vi "virtualinstrument.vi"() -> ()   [LabVIEW 2025]
uses:
  <vilib>/httpClient/LabVIEWHTTPClient.lvlib
  <extravilib>/ChannelInstances/Tag-bool.lvlib
  <vilib>/regexp/Match Regular Expression.xnode
  <vilib>/httpClient/POSTBuffer.vi
  <vilib>/Instr/_visa.llb/VISA Configure Serial Port (Instr).vi
panel:
  out "indexminim":i32
  out "indexmax":i32
  out "humarray":dbl[](array[numeric])
  out "temparray":dbl[](array[numeric])
  out "ppmarray":dbl[](array[numeric])
  out "<JSON>":string[](array[string]) caption="<JSON>Elements"
  in  "Tab Control":enum32{"Page 1"}(tab)
  in  "Select interval":bool
  in  "min":string(combo)
  out "Waveform Chart":dbl[](graph) caption="PPM CHART"
  in  "Select":enum16{"hum", "temp", "ppm"}(ring)
  out "Umiditate":dbl(knob) scale=0.0..100.0
  out "Temperatura":dbl(slide) caption="Thermometer" scale=0.0..100.0
  in  "stop":bool
  in  "Enum":enum16{"PPM", "TEMP", "HUM"}(ring)
  in  "interval \nmasurare[s]":u32=1
  out "XY Graph":cluster{"array":u32[], dbl[]}(graph) caption="PPM GRAPH"
  in  "interval \ntrimitere[s]":u32=1
  out "error out":errorcluster
  out "read buffer":string
  out "ppm":u32(colorbox)
  out "confort termic":dbl
  out "heat index":dbl
  out "ppm":dbl
  in  "Get data from \nspreadsheet":bool
  out "datesarray":timestamp[](array[timestamp]) format="%<%H:%M:%S\n%x>T"
  out "max value":timestamp format="%<%H:%M:%S\n%x>T"
  out "min value":timestamp format="%<%H:%M:%S\n%x>T"
  in  "max":string(combo)
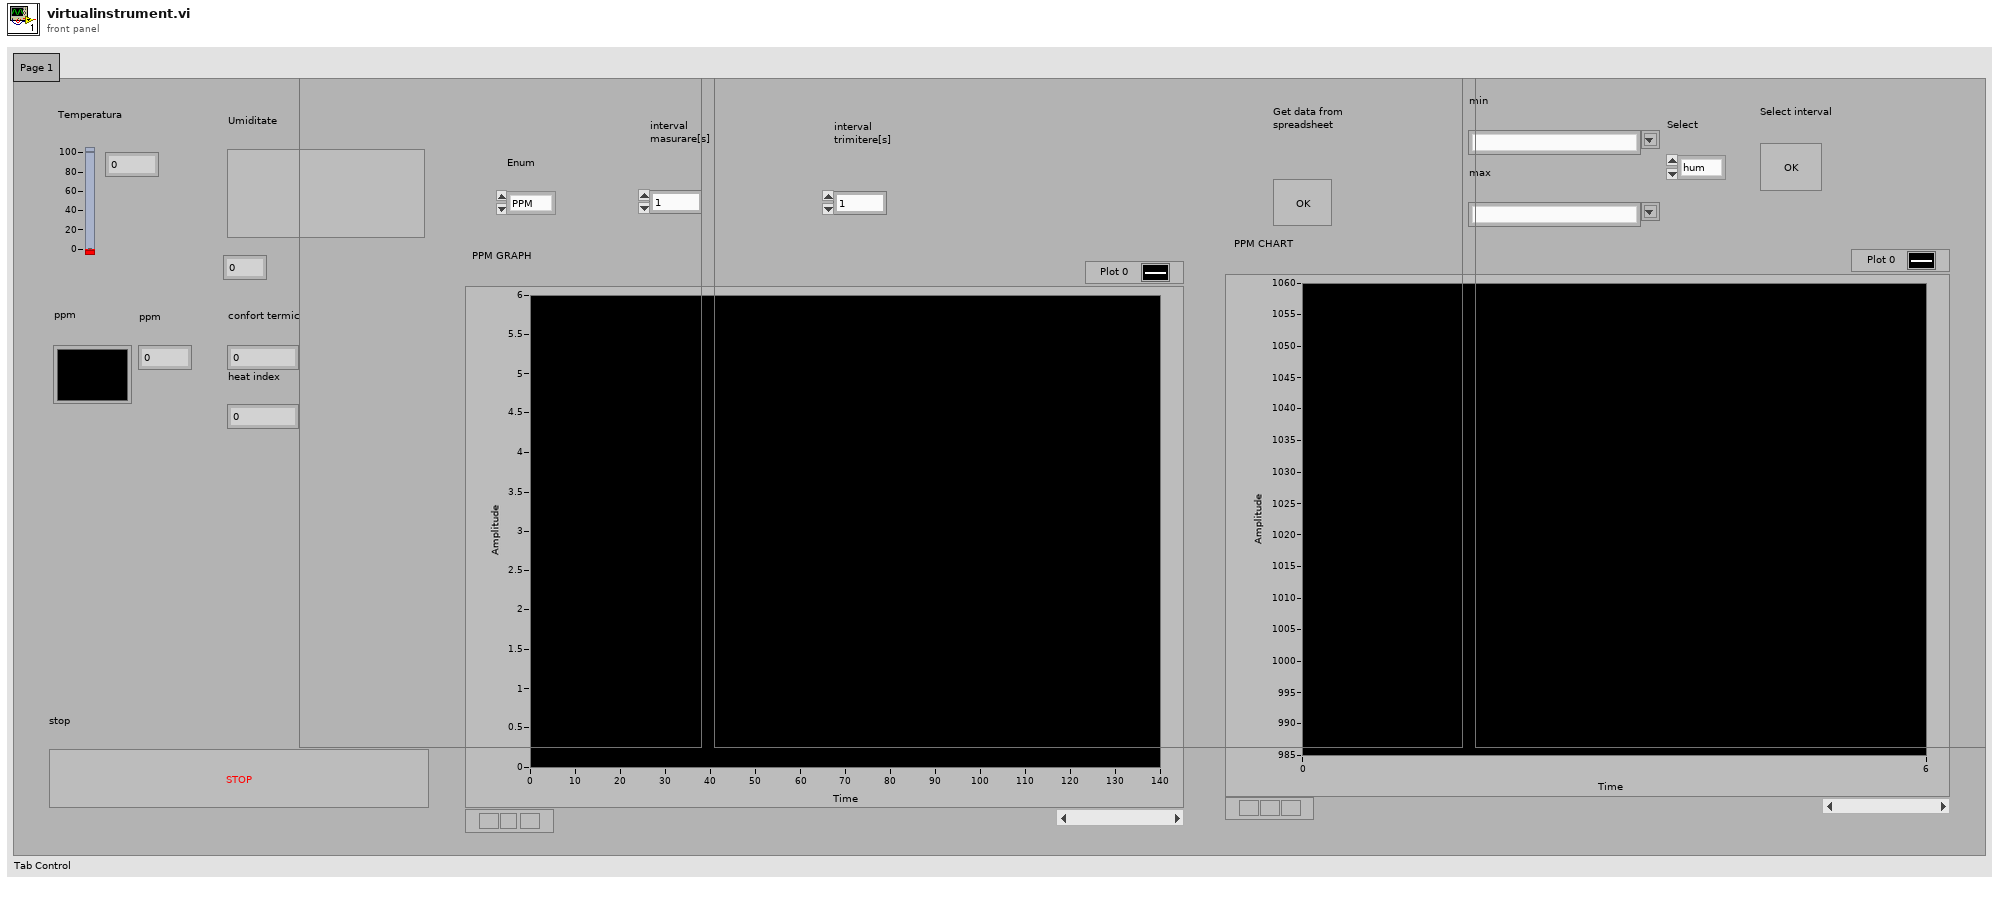
[diagram p1: front panel]
types:
  T1 = typedef "Tag-bool.lvlib/))Channel.ctl" = refnum<queue>
  T2 = enum8{"Enabled", "Disabled", "Disabled and Grayed Out"}
  T3 = typedef "LabVIEWHTTPClient.lvlib/ClientHandle.ctl" = refnum<k1>
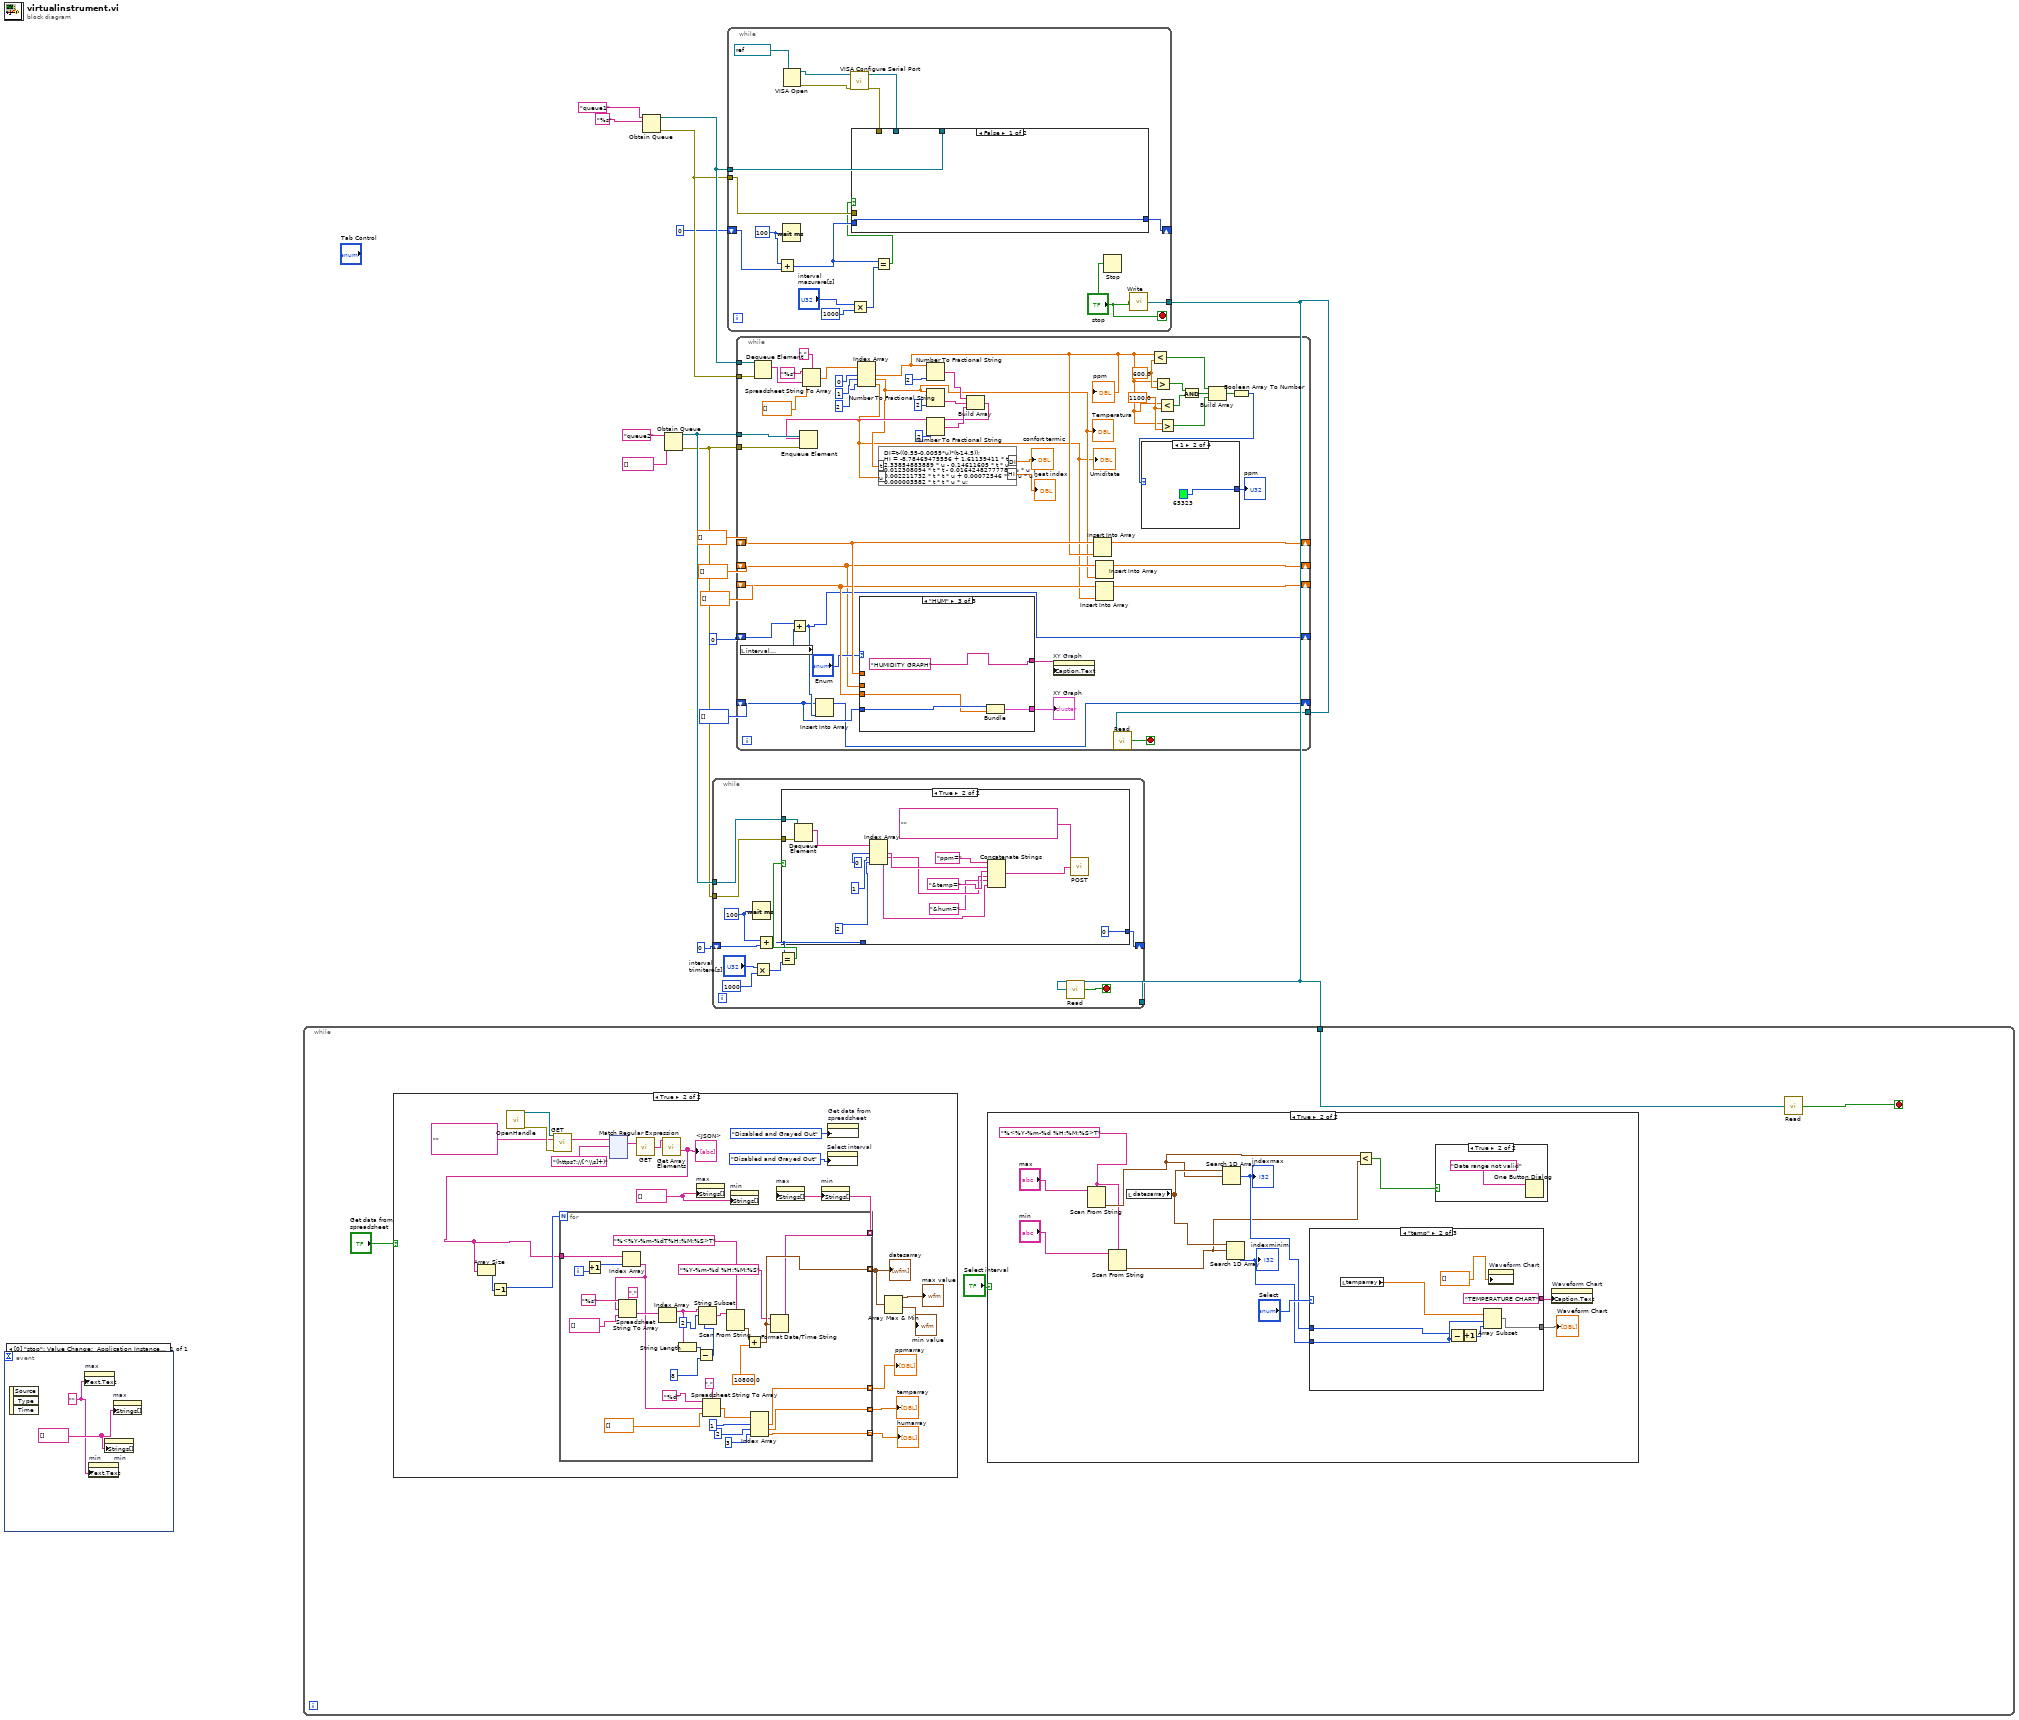
[diagram p0: block diagram]
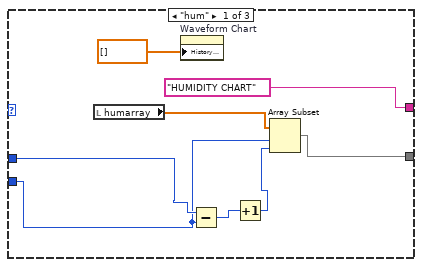
[diagram p3: hidden frame]
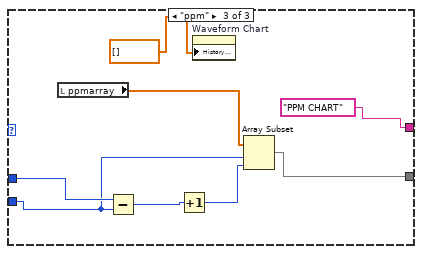
[diagram p4: hidden frame]
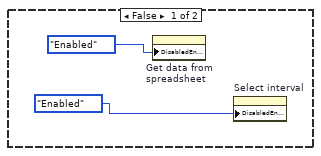
[diagram p6: hidden frame]
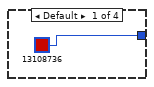
[diagram p8: hidden frame]
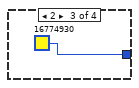
[diagram p9: hidden frame]
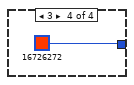
[diagram p10: hidden frame]
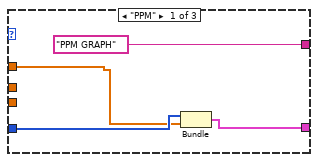
[diagram p11: hidden frame]
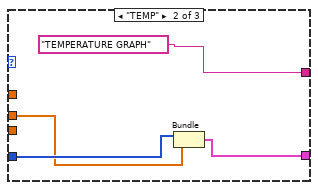
[diagram p12: hidden frame]
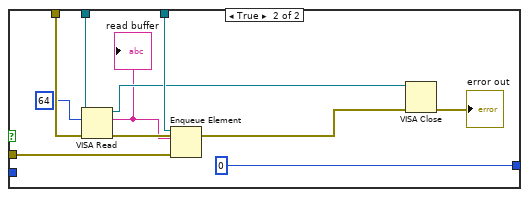
[diagram p13: hidden frame]
diagram:
  n1 = event shown="[0] \"stop\": Value Change;  Application Instance Close" {
    selector: _ -> [_]
    dyn-events: _ -> [_]
    timeout: _ -> [_]
    event "stop": Value Change; Application Instance Close {
      w17 = "" ("Text.Text")
      w18 = string[] []
      n2 = event-data() -> ()  [unwired: 1 in, 3 out]
      n3 = property on="max" class="CmbBox"("Text.Text"=w17) -> ()  [unwired: 2 in, 2 out]
      n4 = property on="min" class="CmbBox"("Text.Text"=w17) -> ()  [unwired: 2 in, 2 out]
      n5 = property on="min" class="CmbBox"("Strings[]"=w18) -> ()  [unwired: 2 in, 2 out]
      n6 = property on="max" class="CmbBox"("Strings[]"=w18) -> ()  [unwired: 2 in, 2 out]
    }
  }
  n7 = Obtain Queue(name (unnamed)="queue1", element data type="%s") -> (queue out=w7:refnum<queue>, error out=w6:errorcluster)  [unwired: 3 in, 1 out]
  n8 = Obtain Queue(name (unnamed)="queue2", element data type=string[] []) -> (queue out=w12:refnum<queue>, error out=w11:errorcluster)  [unwired: 3 in, 1 out]
  n9 = while {
    tunnel: [w35] -> w1
    tunnel: w7 -> [w28]
    tunnel: w6 -> [w27]
    shift-right: [w29] -> _
    shift-left: u32 0 ("y") -> [w26]
    stop <- "stop" stop-if-true
    w30 = u32 100 ("y")
    n10 = Add(x=w30, y=w26) -> (x+y=w22:u32)
    n11 = Wait (ms)(milliseconds to wait=w30) -> ()  [unwired: 1 out]
    n12 = VISA Open(VISA resource name=refnum<visa-resource-name> "COM3") -> (VISA resource name=w33:refnum<visa-resource-name>, error out=w34:errorcluster)  [unwired: 4 in]
    n13 = call-poly "VISA Configure Serial Port"("VISA resource name"=w33, "error in (no error)"=w34) -> ("VISA resource name out"=w19:refnum<visa-resource-name>, "error out"=w20:errorcluster)  [unwired: 12 in]
    n14 = Multiply(x="interval \nmasurare[s]", y=u32 1000) -> (x*y=w23:u32)
    n15 = Equal?(x=w22, y=w23) -> (x = y?=w21:bool)
    n16 = case shown="False" w21 {
      tunnel: [w36 u32 0 ("y")] -> w29
      tunnel: w28 -> [_ w45]
      tunnel: w27 -> [_ w44]
      tunnel: w22 -> [w36 _]
      tunnel: w20 -> [_ w40]
      tunnel: w19 -> [_ w39]
      frame False {
      }
      frame True {
        n17 = VISA Read(VISA resource name=w39, byte count=u32 64, error in (no error)=w40) -> (VISA resource name out=w43:refnum<visa-resource-name>, read buffer=w38:string, error out=w42:errorcluster)  [unwired: 1 out]
        "read buffer" <- w38
        n18 = Enqueue Element(queue=w45, element=w38, error in (no error)=w44) -> ()  [unwired: 1 in, 3 out]
        n19 = VISA Close(VISA resource name=w43, error in (no error)=w42) -> (error out=→"error out":errorcluster)
      }
    }
    n20 = Stop(stop? (T)="stop") -> ()
    n21 = call <extravilib>:"Write.vi"("element"="stop") -> ("channel"=w35:T1)  [unwired: 1 out]
  }
  n22 = while {
    tunnel: w1 -> [w50]
    stop <- w49 stop-if-true
    n23 = case shown="True" "Get data from \nspreadsheet" {
      frame False {
        n24 = property on="Get data from \nspreadsheet" class="Bool"("DisabledEnum"=T2."Enabled" ("Disabled")) -> ()  [unwired: 2 in, 2 out]
        n25 = property on="Select interval" class="Bool"("DisabledEnum"=T2."Enabled" ("Disabled")) -> ()  [unwired: 2 in, 2 out]
      }
      frame True {
        w92 = string[] []
        n26 = call <vilib>:"OpenHandle.vi"() -> ("client handle out"=w109:T3, "error out"=w108:errorcluster)  [unwired: 14 in]
        n27 = call <vilib>:"GET.vi"("client handle"=w109, "url"="", "error in (no error)"=w108) -> ("headers"=w105:string)  [unwired: 9 in, 3 out]
        n28 = xnode ("Match Regular Expression")("input string"=w105, "regular expression"="(https?://[^\\s]+)") -> ("whole match"=w90:string)  [unwired: 4 in, 4 out]
        n29 = call <vilib>:"GET.vi"("url"=w90) -> ("body"=w104:string)  [unwired: 11 in, 3 out]
        n30 = call <vilib>:"Get Array Elements.vi"("JSON"=w104) -> ("<JSON>"=w94:string[])  [unwired: 8 in, 2 out]
        "<JSON>" <- w94
        n31 = Array Size(array=w94) -> (size(s)=w100:i32)
        n32 = Decrement(x=w100) -> (x-1=w99:i32)
        n33 = for {
          N: w99 -> [_]
          tunnel: w94 -> [w138]
          tunnel: [w130] -> w101 mode=indexing
          tunnel: [w120] -> w103 mode=indexing
          tunnel: [w119] -> w102 mode=indexing
          tunnel: [w114] -> w98 mode=indexing
          tunnel: [w110] -> w93 mode=indexing
          i -> [w139]
          n34 = Increment(x=w139) -> (x+1=w133:i32)
          n35 = Index Array(array=w138, index=w133) -> (element=w118:string)
          n36 = Spreadsheet String To Array(delimiter (Tab)=",", format string="%s" ("delimiter (Tab)"), spreadsheet string=w118, array type (2D Dbl)=string[] []) -> (array=w136:string[])
          n37 = Index Array(array=w136) -> (element=w126:string)  [unwired: 1 in]
          n38 = String Length(string=w126) -> (length=w125:i32)
          n39 = Subtract(x=w125, y=8) -> (x-y=w123:i32)
          n40 = String Subset(string=w126, offset (0)=2, length (rest)=w123) -> (substring=w113:string)
          n41 = Spreadsheet String To Array(delimiter (Tab)=",", format string="%d", spreadsheet string=w118, array type (2D Dbl)=dbl[] []) -> (array=w128:dbl[])
          n42 = Scan From String(format string="%<%Y-%m-%dT%H:%M:%S>T", input string=w113) -> (output 1=w115:timestamp)  [unwired: 3 in, 3 out]
          n43 = Add(x=w115, y=10800.0) -> (x+y=w114:timestamp)
          n44 = Index Array(array=w128, index #1=1 ("index"), index #2=2 ("index"), index #3=3 ("index")) -> (element #1=w130:dbl, element #2=w120:dbl, element #3=w119:dbl)
          n45 = Format Date/Time String(time format string (%c)="%Y-%m-%d %H:%M:%S", seconds (now)=w114) -> (date/time string=w110:string)  [unwired: 1 in]
        }
        "ppmarray" <- w101
        "temparray" <- w103
        "humarray" <- w102
        "datesarray" <- w98
        n46 = property on="max" class="CmbBox"("Strings[]"=w92) -> ()  [unwired: 2 in, 2 out]
        n47 = property on="min" class="CmbBox"("Strings[]"=w92) -> ()  [unwired: 2 in, 2 out]
        n48 = property on="max" class="CmbBox"("Strings[]"=w93) -> ()  [unwired: 2 in, 2 out]
        n49 = property on="min" class="CmbBox"("Strings[]"=w93) -> ()  [unwired: 2 in, 2 out]
        n50 = property on="Select interval" class="Bool"("DisabledEnum"=T2."Disabled and Grayed Out" ("Disabled")) -> ()  [unwired: 2 in, 2 out]
        n51 = property on="Get data from \nspreadsheet" class="Bool"("DisabledEnum"=T2."Disabled and Grayed Out" ("Disabled")) -> ()  [unwired: 2 in, 2 out]
        n52 = Array Max & Min(array=w98) -> (max value=→"max value":timestamp, min value=→"min value":timestamp)  [unwired: 2 out]
      }
    }
    n53 = case shown="True" "Select interval" {
      frame False {
      }
      frame True {
        w54 = "%<%Y-%m-%d %H:%M:%S>T" ("format string")
        n54 = Scan From String(format string=w54, input string="max") -> (output 1=w57:timestamp)  [unwired: 3 in, 3 out]
        n55 = Scan From String(format string=w54, input string="min") -> (output 1=w53:timestamp)  [unwired: 3 in, 3 out]
        n56 = local read "datesarray"() -> (w60:timestamp[])
        n57 = Search 1D Array(1D array=w60, element=w57) -> (index of element=w59:i32)  [unwired: 1 in]
        "indexmax" <- w59
        n58 = Search 1D Array(1D array=w60, element=w53) -> (index of element=w58:i32)  [unwired: 1 in]
        "indexminim" <- w58
        n59 = case shown="\"temp\"" "Select" {
          tunnel: w58 -> [w66 w75 w79]
          tunnel: w59 -> [w67 w74 w82]
          tunnel: [w65 w73 w83] -> w61
          tunnel: ["HUMIDITY CHART" ("Caption.Text") "TEMPERATURE CHART" ("Caption.Text") "PPM CHART" ("Caption.Text")] -> w51
          frame "hum" {
            n60 = local read "humarray"() -> (w70:dbl[])
            n61 = property on="Waveform Chart" class="WFChart (strict)"("History Data"=dbl[] []) -> ()  [unwired: 2 in, 2 out]
            n62 = Subtract(x=w67, y=w66) -> (x-y=w69:i32)
            n63 = Increment(x=w69) -> (x+1=w68:i32)
            n64 = Array Subset(array=w70, index=w66, length=w68) -> (w65:dbl[])
          }
          frame "temp" {
            n65 = local read "temparray"() -> (w78:dbl[])
            n66 = Subtract(x=w74, y=w75) -> (x-y=w77:i32)
            n67 = Increment(x=w77) -> (x+1=w76:i32)
            n68 = Array Subset(array=w78, index=w75, length=w76) -> (w73:dbl[])
            n69 = property on="Waveform Chart" class="WFChart (strict)"("History Data"=dbl[] []) -> ()  [unwired: 2 in, 2 out]
          }
          frame "ppm" {
            n70 = local read "ppmarray"() -> (w86:dbl[])
            n71 = Subtract(x=w82, y=w79) -> (x-y=w85:i32)
            n72 = Increment(x=w85) -> (x+1=w84:i32)
            n73 = property on="Waveform Chart" class="WFChart (strict)"("History Data"=dbl[] []) -> ()  [unwired: 2 in, 2 out]
            n74 = Array Subset(array=w86, index=w79, length=w84) -> (w83:dbl[])
          }
        }
        "Waveform Chart" <- w61
        n75 = Less?(x=w57, y=w53) -> (x < y?=w52:bool)
        n76 = case shown="True" w52 {
          frame False {
          }
          frame True {
            n77 = One Button Dialog(message="Date range not valid") -> ()  [unwired: 1 in, 1 out]
          }
        }
        n78 = property on="Waveform Chart" class="WFChart (strict)"("Caption.Text"=w51) -> ()  [unwired: 2 in, 2 out]
      }
    }
    n79 = call <extravilib>:"Read.vi"("channel"=w50) -> ("element"=w49:bool)  [unwired: 1 in, 1 out]
  }
  n80 = while {
    tunnel: w12 -> [w258]
    tunnel: w11 -> [w257]
    tunnel: w1 -> [w268]
    shift-right: [w259] -> _
    shift-left: u32 0 ("y") -> [w263]
    stop <- w267 stop-if-true
    w266 = u32 100 ("y")
    n81 = Wait (ms)(milliseconds to wait=w266) -> ()  [unwired: 1 out]
    n82 = Multiply(x="interval \ntrimitere[s]", y=u32 1000) -> (x*y=w264:u32)
    n83 = Add(x=w266, y=w263) -> (x+y=w260:u32)
    n84 = Equal?(x=w260, y=w264) -> (x = y?=w261:bool)
    n85 = case shown="True" w261 {
      tunnel: w260 -> [w269 _]
      tunnel: [w269 u32 0 ("y")] -> w259
      tunnel: w258 -> [_ w279]
      tunnel: w257 -> [_ w278]
      frame False {
      }
      frame True {
        n86 = Dequeue Element(queue=w279, error in (no error)=w278) -> (element=w277:string[])  [unwired: 1 in, 3 out]
        n87 = Index Array(array=w277, index #1=0 ("index"), index #2=1 ("index"), index #3=2 ("index")) -> (element #1=w281:string, element #2=w273:string, element #3=w271:string)
        n88 = Concatenate Strings("ppm=" ("string"), w281, "&temp=" ("string"), w273, "&hum=" ("string"), w271) -> (w270:string)
        n89 = call-poly <vilib>:"POST.vi"("url"="", "buffer"=w270) -> ()  [unwired: 10 in, 4 out]
      }
    }
    n90 = call <extravilib>:"Read.vi"("channel"=w268) -> ("element"=w267:bool)  [unwired: 1 in, 1 out]
  }
  n91 = while {
    tunnel: w7 -> [w326]
    tunnel: w6 -> [w325]
    tunnel: w12 -> [w323]
    tunnel: w11 -> [w322]
    shift-right: [w317] -> _
    shift-left: dbl[] [] -> [w314]
    shift-right: [w316] -> _
    shift-left: dbl[] [] -> [w306]
    shift-right: [w315] -> _
    shift-left: dbl[] [] -> [w313]
    tunnel: w1 -> [w311]
    shift-right: [w308] -> _
    shift-left: 0 -> [w310]
    shift-right: [w304] -> _
    shift-left: u32[] [] ("array") -> [w305]
    stop <- w290 stop-if-true
    w299 = 1100.0 ("y")
    w292 = 600.0 ("y")
    n92 = local read "interval \nmasurare[s]"() -> (w309:u32)
    n93 = Dequeue Element(queue=w326, error in (no error)=w325) -> (element=w324:string)  [unwired: 1 in, 3 out]
    n94 = Add(x=w310, y=w309) -> (x+y=w308:u32)
    n95 = Spreadsheet String To Array(delimiter (Tab)=",", format string="%s", spreadsheet string=w324, array type (2D Dbl)=dbl[] []) -> (array=w327:dbl[])
    n96 = Insert Into Array(array=w305, new element=w308) -> (w304:u32[])  [unwired: 1 in]
    n97 = Index Array(array=w327, index #1=0 ("index"), index #2=1 ("index"), index #3=2 ("index")) -> (element #1=w291:dbl, element #2=w287:dbl, element #3=w286:dbl)
    "Temperatura" <- w287
    "Umiditate" <- w286
    "ppm" <- w291
    n98 = case shown="\"HUM\"" "Enum" {
      tunnel: w314 -> [w340 _ _]
      tunnel: w306 -> [_ w344 _]
      tunnel: w313 -> [_ _ w348]
      tunnel: w305 -> [w342 w346 w349]
      tunnel: [w341 w345 w350] -> w307
      tunnel: ["PPM GRAPH" ("Label.Text") "TEMPERATURE GRAPH" ("Label.Text") "HUMIDITY GRAPH" ("Label.Text")] -> w285
      frame "PPM" {
        n99 = Bundle("array"=w342, w340) -> (w341:cluster{"array":u32[], dbl[]})  [unwired: 1 in]
      }
      frame "TEMP" {
        n100 = Bundle("array"=w346, w344) -> (w345:cluster{"array":u32[], dbl[]})  [unwired: 1 in]
      }
      frame "HUM" {
        n101 = Bundle("array"=w349, w348) -> (w350:cluster{"array":u32[], dbl[]})  [unwired: 1 in]
      }
    }
    "XY Graph" <- w307
    n102 = formula code="DI=t-((0.55-0.0055*u)*(t-14.5));\nHI = -8.78469475556 + 1.61139411 * t + 2.33854883889 * u - 0.14611605 * t * u - 0.012308094 * t * t - 0.0164248277778 * u * u + 0.002211732 * t * t * u + 0.00072546 * t * u * u - 0.000003582 * t * t * u * u;"("t"=w287, "u"=w286) -> ("DI"=→"confort termic":dbl, "HI"=→"heat index":dbl)
    n103 = Number To Fractional String(number=w291, precision (6)=i16 2) -> (F-format string=w321:string)  [unwired: 2 in]
    n104 = Number To Fractional String(number=w287, precision (6)=i16 2) -> (F-format string=w320:string)  [unwired: 2 in]
    n105 = Number To Fractional String(number=w286, precision (6)=i16 2) -> (F-format string=w319:string)  [unwired: 2 in]
    n106 = Build Array(w321, w320, w319) -> (w318:string[])
    n107 = Enqueue Element(queue=w323, element=w318, error in (no error)=w322) -> ()  [unwired: 1 in, 3 out]
    n108 = property on="XY Graph" class="XYGraph (strict)"("Caption.Text"=w285) -> ()  [unwired: 2 in, 2 out]
    n109 = Insert Into Array(array=w314, new element=w291) -> (w317:dbl[])  [unwired: 1 in]
    n110 = Insert Into Array(array=w306, new element=w287) -> (w316:dbl[])  [unwired: 1 in]
    n111 = Insert Into Array(array=w313, new element=w286) -> (w315:dbl[])  [unwired: 1 in]
    n112 = call <extravilib>:"Read.vi"("channel"=w311) -> ("element"=w290:bool)  [unwired: 1 in, 1 out]
    n113 = Less?(x=w291, y=w292) -> (x < y?=w298:bool)
    n114 = Greater?(x=w291, y=w292) -> (0:w301:bool)
    n115 = Less?(x=w291, y=w299) -> (x < y?=w300:bool)
    n116 = Greater?(x=w291, y=w299) -> (0:w296:bool)
    n117 = And(x=w301, y=w300) -> (x .and. y?=w297:bool)
    n118 = Build Array(w298, w297, w296) -> (w295:bool[])
    n119 = Boolean Array To Number(Boolean array=w295) -> (number=w294:u32)
    n120 = case shown="1" w294 {
      tunnel: [u32 13108736 u32 65323 u32 16774930 u32 16726272] -> w293
      frame Default {
      }
      frame 1 {
      }
      frame 2 {
      }
      frame 3 {
      }
    }
    "ppm" <- w293
  }
